vi "PV ActiveLine - UnderrangeControl.vi"(7 "W/R":bool, 8 "Fehler (Eingang)":errorcluster, 10 "Sensor 1 Set":u8(ring) items=["off", "on"], 11 "Referenz in":refnum<visa-resource-name>) -> (0 "Cluster (Ausgang)":errorcluster, 2 "Sensor 1 Get":u8(ring) items=["off", "on"], 3 "Referenz out":refnum<visa-resource-name>)   [LabVIEW 2013, in "PV ActiveLine.lvlib"]
doc: "PUC - Underrange Control\n\nTransmit: PUC [,a]\nReceive: a\n\na =\n0 –> Off (default)\n1 –> On"
uses:
  <instrlib>/PV ActiveLine/PV ActiveLine.lvlib
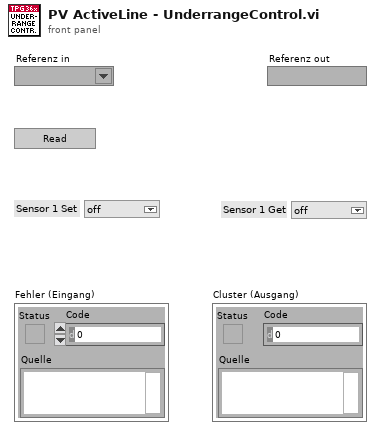
[diagram p1: front panel]
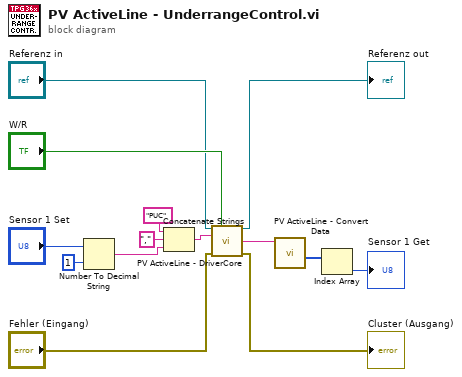
[diagram p0: block diagram]
diagram:
  n1 = Number To Decimal String(number="Sensor 1 Set", width (-)=i16 1 ("Breite (-)")) -> (decimal integer string=w3:string)
  n2 = Concatenate Strings("PUC", "," ("String"), w3) -> (w12:string)
  n3 = call <instrlib>:"PV ActiveLine - DriverCore.vi"("Referenz in"="Referenz in", "Write/Read"="W/R", "Command"=w12, "Fehler (Eingang)"="Fehler (Eingang)") -> ("Referenz out"=→"Referenz out":refnum<visa-resource-name>, "String Out"=w7:string, "Cluster (Ausgang)"=→"Cluster (Ausgang)":errorcluster)  [unwired: 9 in]
  n4 = call <instrlib>:"PV ActiveLine - Convert Data.vi"("String in"=w7) -> ("Integer Out"=w6:i32[])  [unwired: 7 in, 3 out]
  n5 = Index Array(array=w6) -> (element=→"Sensor 1 Get":i32)  [unwired: 1 in]
